vi "Close Thor WP.vi"(3 "error in (no error)":errorcluster, 5 "input Kcube refnum cluster":T1) -> (0 "error out":errorcluster)   [LabVIEW 2015]
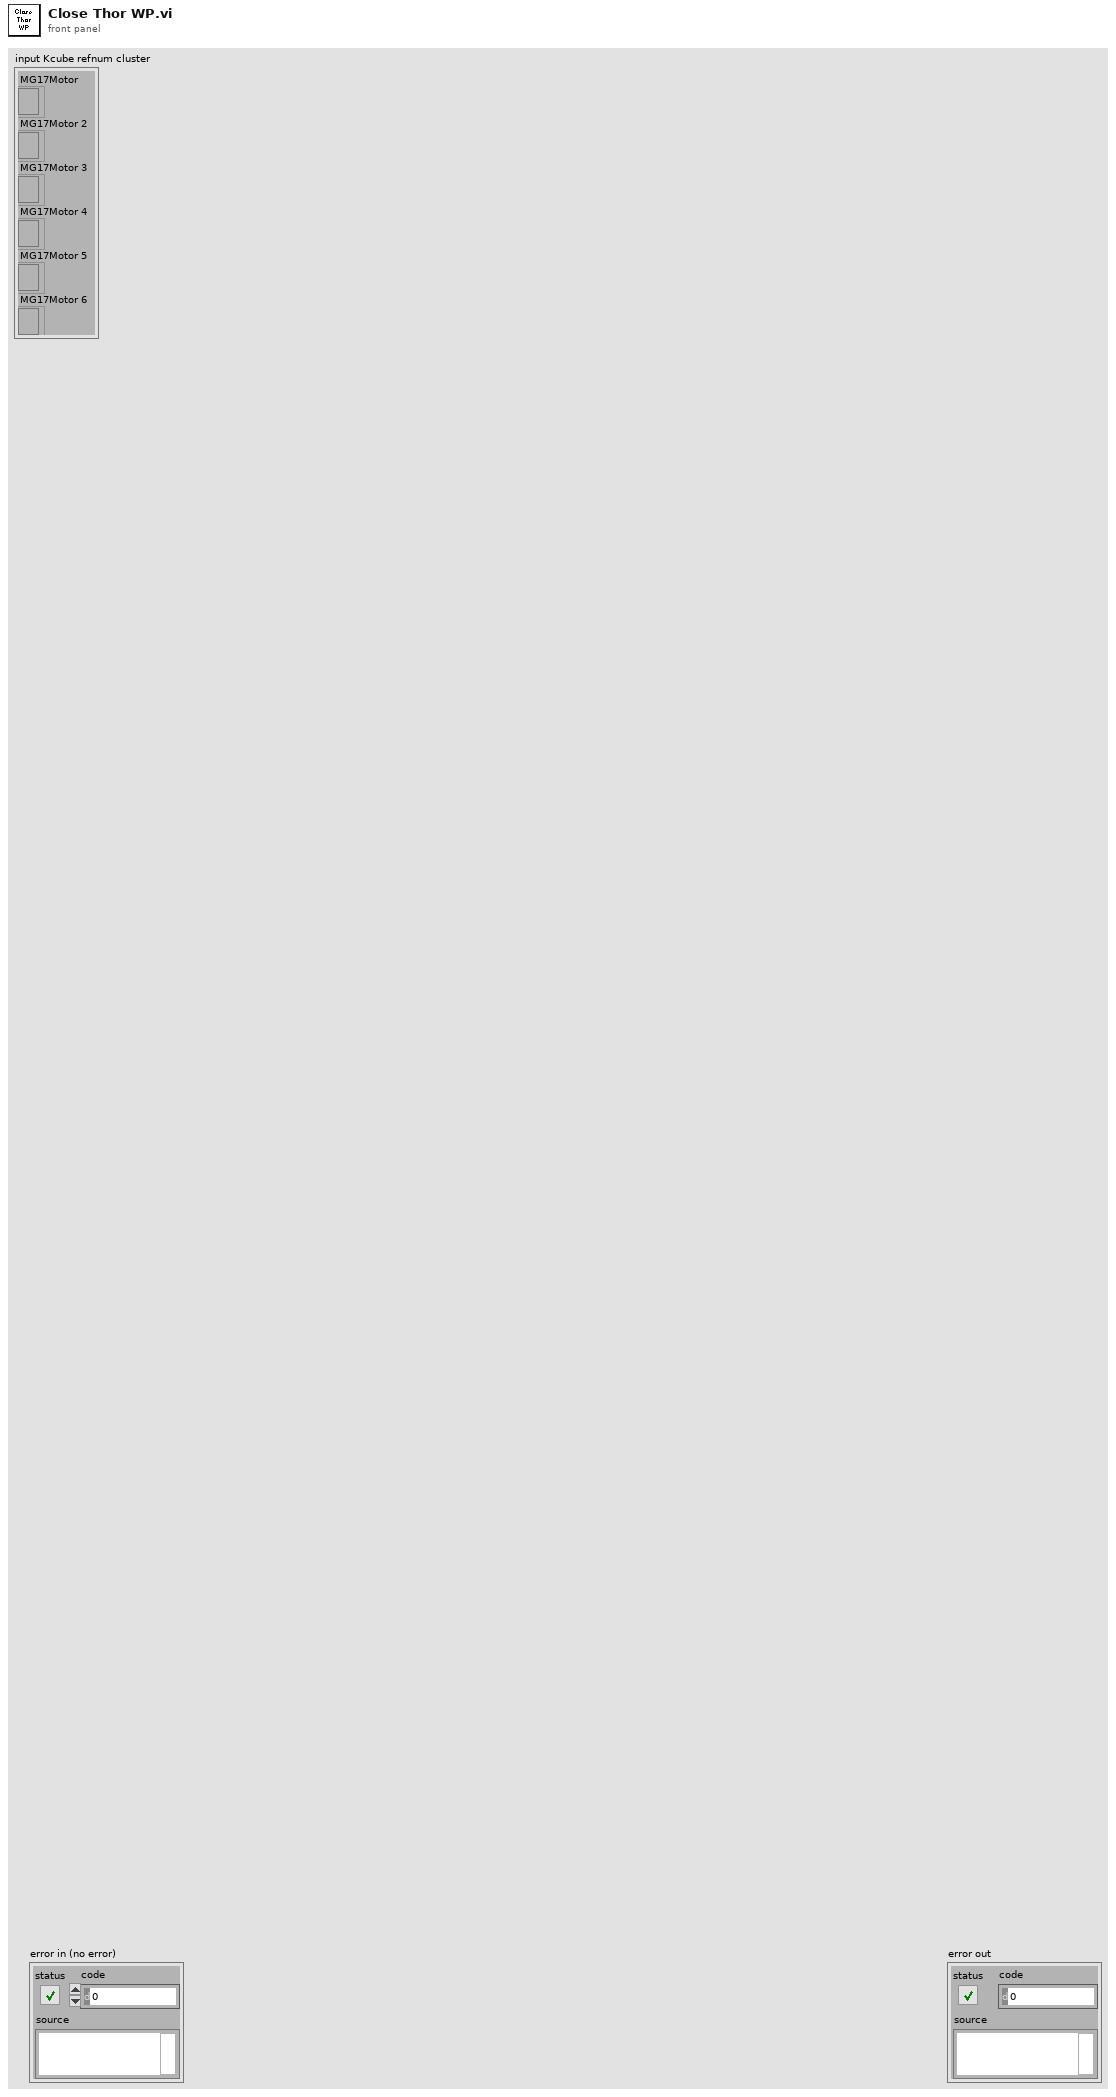
[diagram p1: front panel]
types:
  T1 = cluster{"MG17Motor":refnum<k7>, "MG17Motor 2":refnum<k7>, "MG17Motor 3":refnum<k7>, "MG17Motor 4":refnum<k7>, "MG17Motor 5":refnum<k7>, "MG17Motor 6":refnum<k7>}
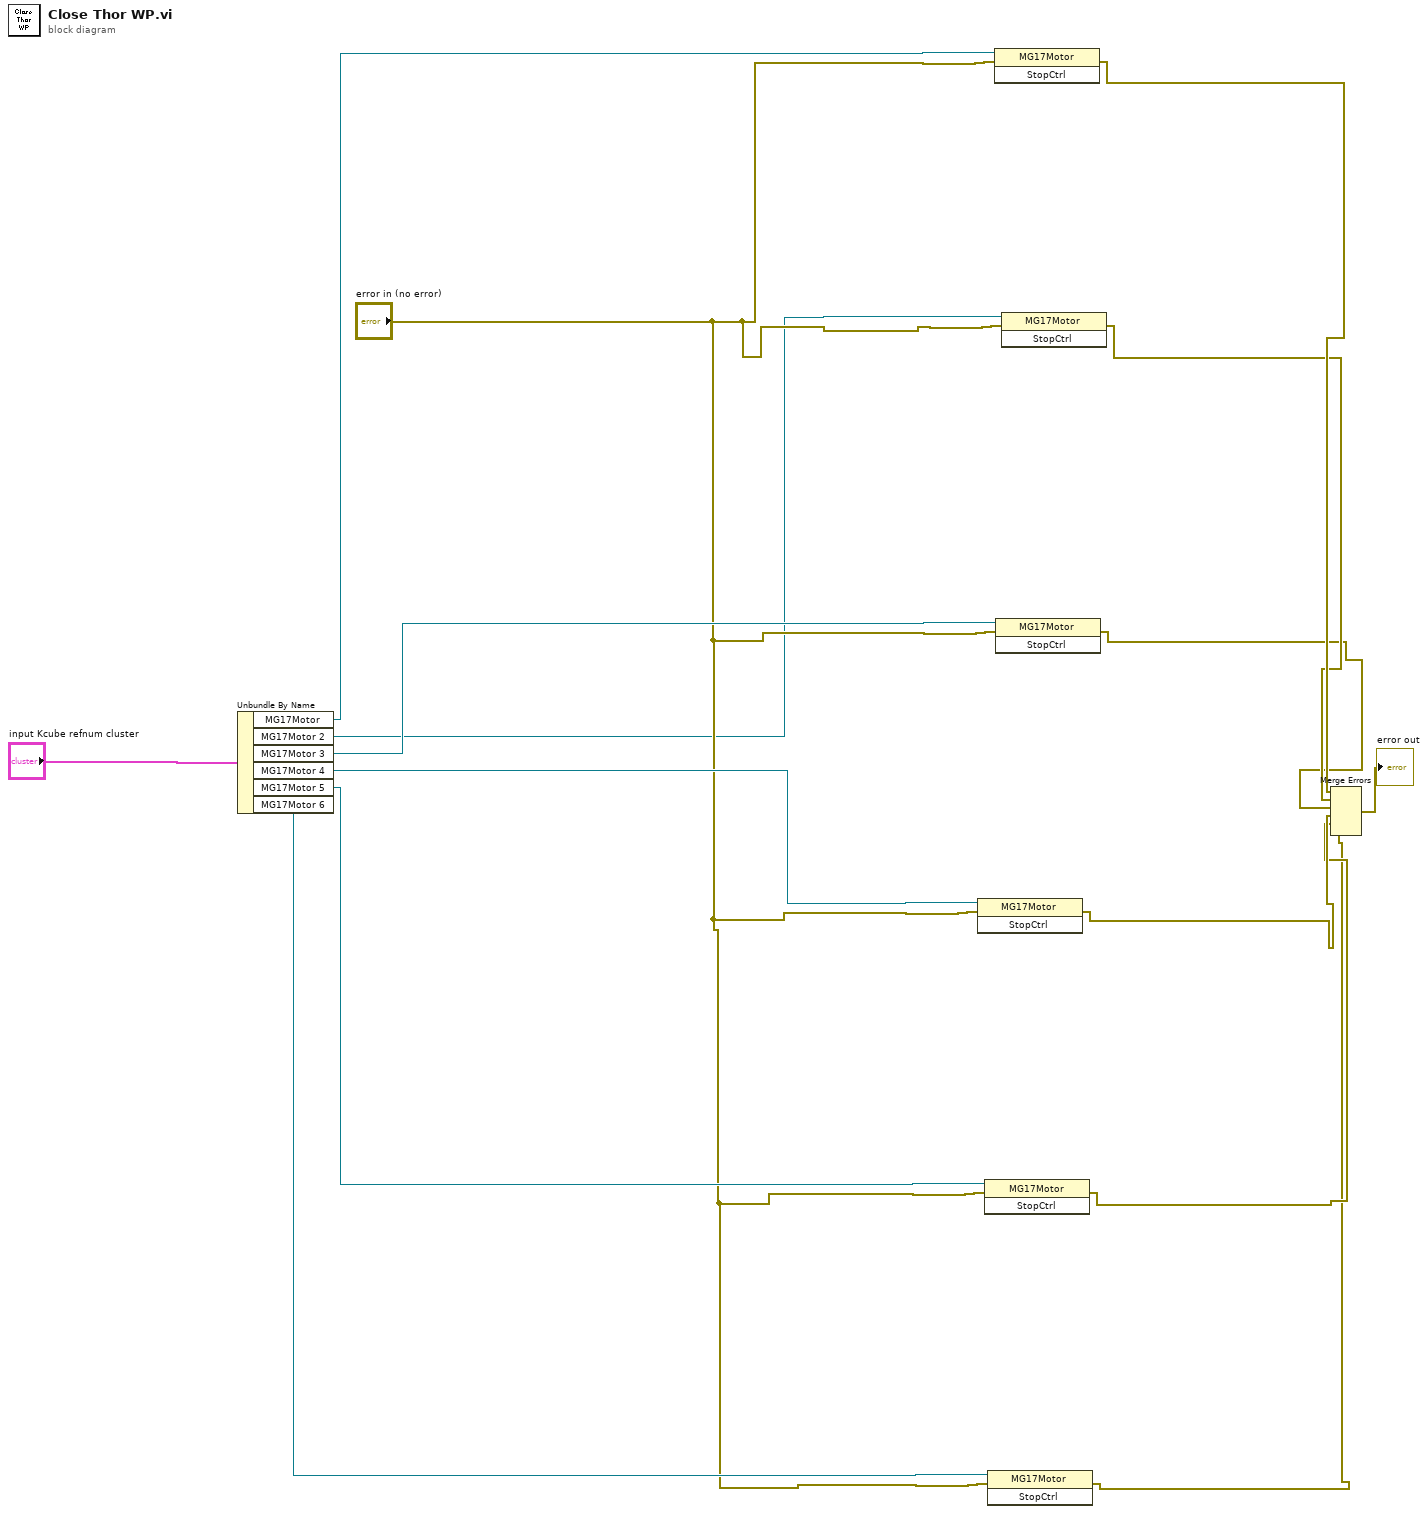
[diagram p0: block diagram]
diagram:
  n1 = Unbundle By Name("input Kcube refnum cluster") -> ("MG17Motor"=w7:refnum<k7>, "MG17Motor 2"=w1:refnum<k7>, "MG17Motor 3"=w3:refnum<k7>, "MG17Motor 4"=w4:refnum<k7>, "MG17Motor 5"=w5:refnum<k7>, "MG17Motor 6"=w6:refnum<k7>)
  n2 = invoke class="MG17Motor" method="StopCtrl"(reference=w4, error in="error in (no error)") -> (error out=w10:errorcluster)  [unwired: 1 in, 2 out]
  n3 = invoke class="MG17Motor" method="StopCtrl"(reference=w5, error in="error in (no error)") -> (error out=w9:errorcluster)  [unwired: 1 in, 2 out]
  n4 = invoke class="MG17Motor" method="StopCtrl"(reference=w6, error in="error in (no error)") -> (error out=w8:errorcluster)  [unwired: 1 in, 2 out]
  n5 = invoke class="MG17Motor" method="StopCtrl"(reference=w7, error in="error in (no error)") -> (error out=w13:errorcluster)  [unwired: 1 in, 2 out]
  n6 = invoke class="MG17Motor" method="StopCtrl"(reference=w3, error in="error in (no error)") -> (error out=w11:errorcluster)  [unwired: 1 in, 2 out]
  n7 = invoke class="MG17Motor" method="StopCtrl"(reference=w1, error in="error in (no error)") -> (error out=w12:errorcluster)  [unwired: 1 in, 2 out]
  n8 = Merge Errors(w13, w12, w11, w10, w9, w8) -> (→"error out":errorcluster)
